vi "Interface_Asset_Map Control.vi"(8 "error in (no error)":errorcluster, 11 "Load in":refnum<class "Load.lvclass">) -> (0 "error out":errorcluster, 3 "Load out":refnum<class "Load.lvclass">)   [LabVIEW 2015, in "Load.lvclass"]
uses:
  Load.lvclass
  Interface_Asset/Interface_Asset.lvclass
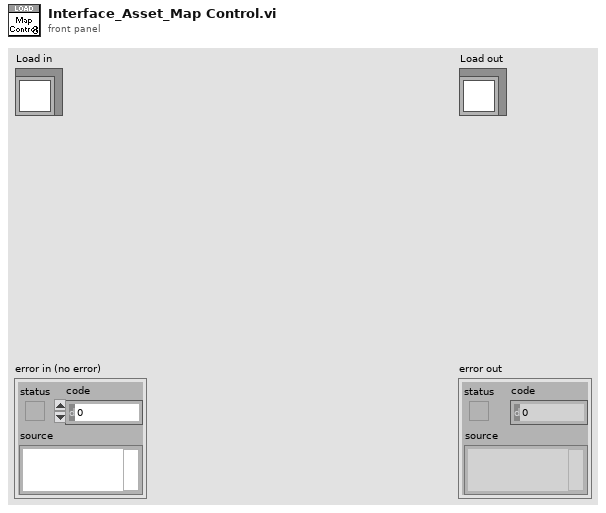
[diagram p1: front panel]
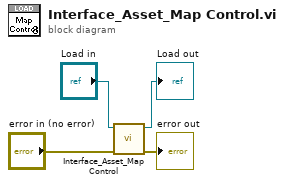
[diagram p0: block diagram]
diagram:
  n1 = call-parent "Interface_Asset_Map Control.vi"("error in (no error)"="error in (no error)", "Interface_Asset in"="Load in") -> ("error out"=→"error out":errorcluster, "Interface_Asset out"=→"Load out":refnum<class "Load.lvclass">)  [unwired: 8 in]
